vi "K6221_sweep.vi"(0 "VISA resource name":refnum<visa-resource-name>="GPIB0::10::INSTR", 1 "Stop mA":dbl=1e-05 min=-0.007 max=7.0 format="%^.3e", 2 "Start mA":dbl=0.1 min=-0.105 max=7.0 format="%^.3e", 3 "error in":errorcluster, 4 "Compliance Voltage":dbl=10.0 format="%.3f", 6 "Time min":dbl=0.1 format="%.3f", 7 "mode":enum16{"linear", "log", "custom"}(ring)) -> (5 "VISA resource name 2":refnum<visa-resource-name>, 8 "error out":errorcluster)   [LabVIEW 2019]
panel:
  in  "Compliance Voltage 2":dbl=10.0 format="%.3f"
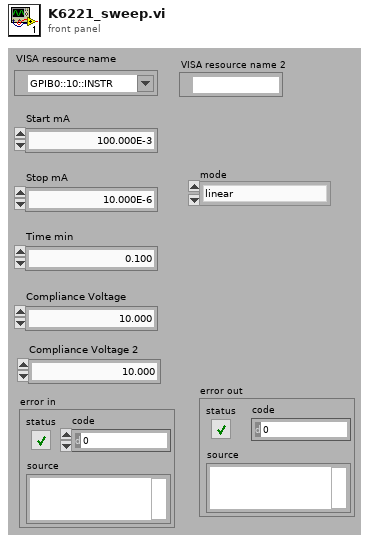
[diagram p1: front panel]
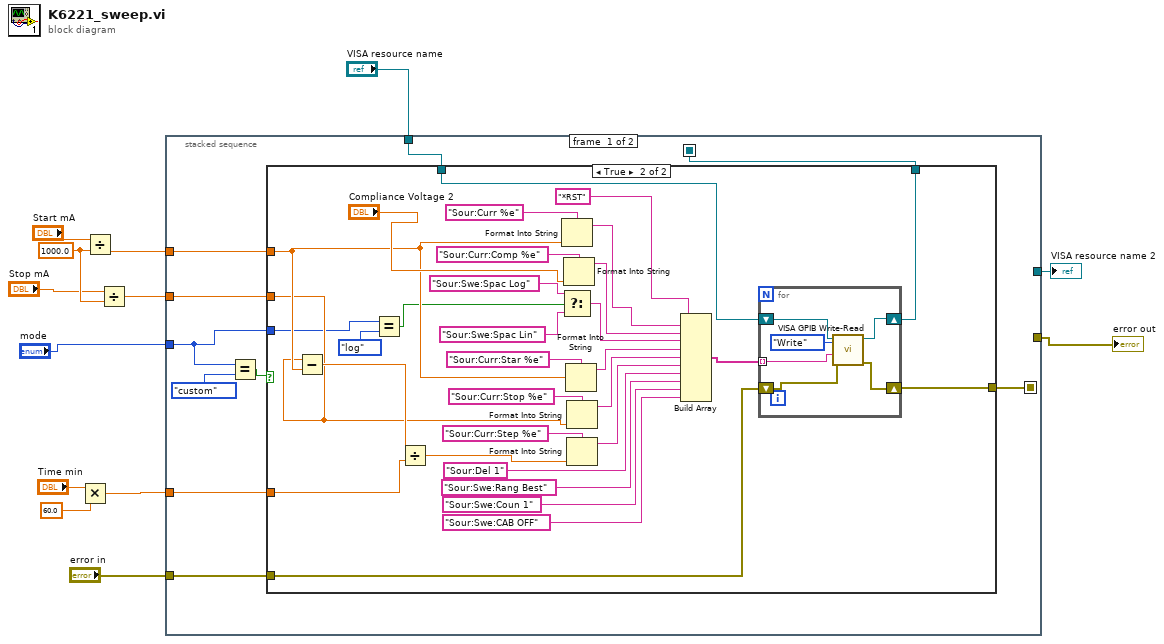
[diagram p0: block diagram]
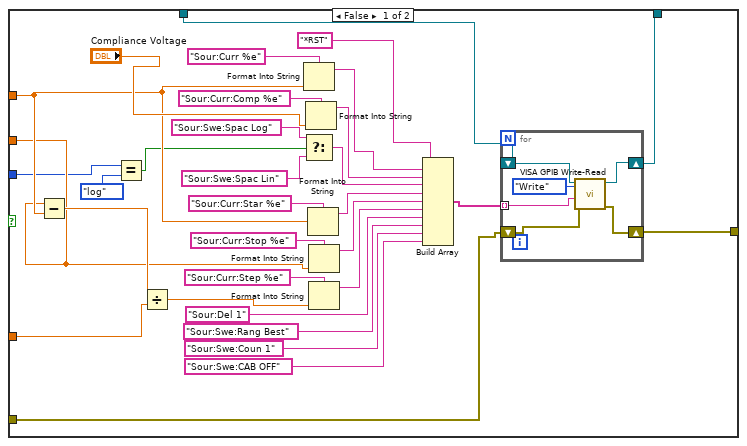
[diagram p2: hidden frame]
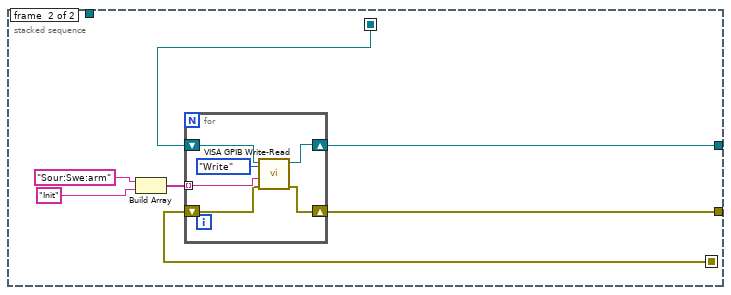
[diagram p3: hidden frame]
diagram:
  w12 = 1000.0 ("y")
  n1 = Multiply(x="Time min", y=60.0) -> (x*y=w5:dbl)
  n2 = Divide(x="Start mA", y=w12) -> (x/y=w9:dbl)
  n3 = Divide(x="Stop mA", y=w12) -> (x/y=w8:dbl)
  n4 = stacked-sequence {
    seq-local: [w22 _] -> [_ w103]
    seq-local: [w15 _] -> [_ w102]
    tunnel: "VISA resource name" -> [w23 _]
    tunnel: w9 -> [w21 _]
    tunnel: w8 -> [w20 _]
    tunnel: w5 -> [w19 _]
    tunnel: "mode" -> [w17 _]
    tunnel: [_ w101] -> w3
    tunnel: [_ w100] -> w2
    tunnel: "error in" -> [w14 _]
    frame #0 {
      n5 = Equal?(x=w17, y=enum16{"linear", "log", "custom"}."custom" ("Enum")) -> (x = y?=w16:bool)
      n6 = case shown="True" w16 {
        tunnel: w23 -> [w33 w71]
        tunnel: [w32 w70] -> w22
        tunnel: w21 -> [w31 w69]
        tunnel: w20 -> [w30 w68]
        tunnel: w19 -> [w29 w67]
        tunnel: w17 -> [w28 w66]
        tunnel: [w25 w63] -> w15
        tunnel: w14 -> [w24 w62]
        frame False {
          n7 = Subtract(x=w30, y=w31) -> (x-y=w55:dbl)
          n8 = Equal?(x=w28, y=enum16{"linear", "log", "custom"}."log" ("Enum")) -> (x = y?=w26:bool)
          n9 = Divide(x=w55, y=w29) -> (x/y=w54:dbl)
          n10 = Format Into String(format string="Sour:Curr %e", w31) -> (resulting string=w41:string)  [unwired: 2 in, 1 out]
          n11 = Select(t="Sour:Swe:Spac Log", s=w26, f="Sour:Swe:Spac Lin") -> (s? t:f=w43:string)
          n12 = Format Into String(format string="Sour:Curr:Comp %e", "Compliance Voltage") -> (resulting string=w42:string)  [unwired: 2 in, 1 out]
          n13 = Format Into String(format string="Sour:Curr:Star %e", w31) -> (resulting string=w44:string)  [unwired: 2 in, 1 out]
          n14 = Format Into String(format string="Sour:Curr:Stop %e", w30) -> (resulting string=w45:string)  [unwired: 2 in, 1 out]
          n15 = Format Into String(format string="Sour:Curr:Step %e", w54) -> (resulting string=w46:string)  [unwired: 2 in, 1 out]
          n16 = Build Array("*RST", w41, w42, w43, w44, w45, w46, "Sour:Del 1", "Sour:Swe:Rang Best", "Sour:Swe:Coun 1", "Sour:Swe:CAB OFF") -> (w51:string[])
          n17 = for {
            tunnel: w51 -> [w60] mode=indexing
            shift-right: [w58] -> w25
            shift-left: w33 -> [w59]
            shift-right: [w57] -> w32
            shift-left: w24 -> [w56]
            n18 = call "VISA GPIB Write-Read.vi"("error in (no error)"=w56, "Command"=w60, "Action"=enum16{"Write", "Read", "Write & Read"}."Write", "VISA resource name"=w59) -> ("error out"=w57:errorcluster, "dup VISA Session"=w58:refnum<visa-resource-name>)  [unwired: 4 in, 2 out]
          }
        }
        frame True {
          n19 = Subtract(x=w68, y=w69) -> (x-y=w93:dbl)
          n20 = Equal?(x=w66, y=enum16{"linear", "log", "custom"}."log" ("Enum")) -> (x = y?=w64:bool)
          n21 = Divide(x=w93, y=w67) -> (x/y=w92:dbl)
          n22 = Format Into String(format string="Sour:Curr %e", w69) -> (resulting string=w79:string)  [unwired: 2 in, 1 out]
          n23 = Select(t="Sour:Swe:Spac Log", s=w64, f="Sour:Swe:Spac Lin") -> (s? t:f=w81:string)
          n24 = Format Into String(format string="Sour:Curr:Comp %e", "Compliance Voltage 2") -> (resulting string=w80:string)  [unwired: 2 in, 1 out]
          n25 = Format Into String(format string="Sour:Curr:Star %e", w69) -> (resulting string=w82:string)  [unwired: 2 in, 1 out]
          n26 = Format Into String(format string="Sour:Curr:Stop %e", w68) -> (resulting string=w83:string)  [unwired: 2 in, 1 out]
          n27 = Format Into String(format string="Sour:Curr:Step %e", w92) -> (resulting string=w84:string)  [unwired: 2 in, 1 out]
          n28 = Build Array("*RST", w79, w80, w81, w82, w83, w84, "Sour:Del 1", "Sour:Swe:Rang Best", "Sour:Swe:Coun 1", "Sour:Swe:CAB OFF") -> (w89:string[])
          n29 = for {
            tunnel: w89 -> [w98] mode=indexing
            shift-right: [w96] -> w63
            shift-left: w71 -> [w97]
            shift-right: [w95] -> w70
            shift-left: w62 -> [w94]
            n30 = call "VISA GPIB Write-Read.vi"("error in (no error)"=w94, "Command"=w98, "Action"=enum16{"Write", "Read", "Write & Read"}."Write", "VISA resource name"=w97) -> ("error out"=w95:errorcluster, "dup VISA Session"=w96:refnum<visa-resource-name>)  [unwired: 4 in, 2 out]
          }
        }
      }
    }
    frame #1 {
      n31 = Build Array("Sour:Swe:arm", "Init") -> (w106:string[])
      n32 = for {
        tunnel: w106 -> [w111] mode=indexing
        shift-right: [w109] -> w101
        shift-left: w102 -> [w110]
        shift-right: [w107] -> w100
        shift-left: w103 -> [w108]
        n33 = call "VISA GPIB Write-Read.vi"("error in (no error)"=w108, "Command"=w111, "Action"=enum16{"Write", "Read", "Write & Read"}."Write", "VISA resource name"=w110) -> ("error out"=w107:errorcluster, "dup VISA Session"=w109:refnum<visa-resource-name>)  [unwired: 4 in, 2 out]
      }
    }
  }
  "VISA resource name 2" <- w3
  "error out" <- w2
